vi "C(i,x,y) T-sum coefficient.vi"(8 "Error In":errorcluster, 9 "y":dbl, 10 "x":dbl, 11 "i":i32) -> (0 "Error Out":errorcluster, 3 "C(i, x, y)":dbl)   [LabVIEW 2021, in "Math.lvlib"]
uses:
  Math.lvlib
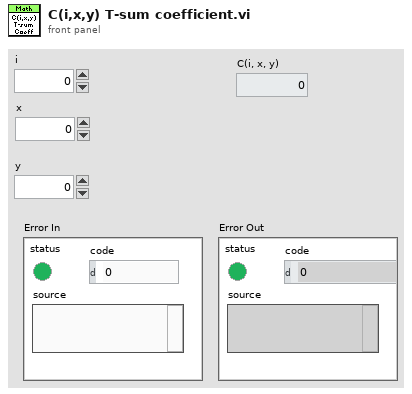
[diagram p1: front panel]
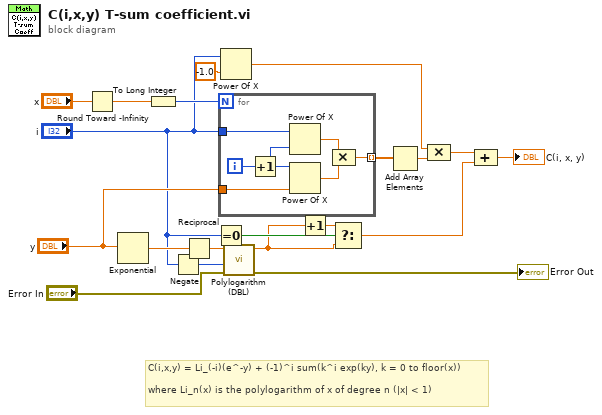
[diagram p0: block diagram]
diagram:
  # "C(i,x,y) = Li_(-i)(e^-y) + (-1)^i sum(k^i exp(ky), k = 0 to floor(x))\n\nwhere Li_n(x) is the polylogarithm of x of degree n (|x| < 1)"
  n1 = Round Toward -Infinity(1:"x") -> (0:w17:dbl)
  n2 = Exponential(1:"y") -> (0:w20:dbl)
  n3 = To Long Integer(number=w17) -> (32bit integer=w16:i32)
  n4 = Negate(x="i") -> (-x=w6:i32)
  n5 = Reciprocal(x=w20) -> (1/x=w15:dbl)
  n6 = Equal To 0?(x="i") -> (x = 0?=w3:bool)
  n7 = for {
    N: w16 -> [_]
    tunnel: "y" -> [w26]
    tunnel: "i" -> [w24]
    tunnel: [w21] -> w13 mode=indexing
    i -> [w27]
    n8 = Increment(x=w27) -> (x+1=w25:i32)
    n9 = Power Of X(1:w25, 2:w24) -> (0:w23:dbl)
    n10 = Power Of X(1:w26, 2:w25) -> (0:w22:dbl)
    n11 = Compound Arithmetic op=MULTIPLY(w23, w22) -> (w21:dbl)
  }
  n12 = Power Of X(1:-1.0 ("x"), 2:"i") -> (0:w10:dbl)
  n13 = call "Polylogarithm (DBL).vi"("Error In"="Error In", "n"=w6, "z"=w15) -> ("Error Out"=→"Error Out":errorcluster, "Li_n(z)"=w2:dbl)  [unwired: 5 in, 2 out]
  n14 = Increment(x=w2) -> (x+1=w1:dbl)
  n15 = Select(t=w1, s=w3, f=w2) -> (s? t:f=w4:dbl)
  n16 = Add Array Elements(numeric array=w13) -> (sum=w12:dbl)
  n17 = Compound Arithmetic op=MULTIPLY(w10, w12) -> (w9:dbl)
  n18 = Compound Arithmetic op=ADD(w9, w4) -> (→"C(i, x, y)":dbl)
